vi "closeSine.vi"(8 "error in (no error)":errorcluster, 11 "VISA Refnum in":refnum<visa-resource-name>) -> (0 "error out":errorcluster)   [LabVIEW 2012]
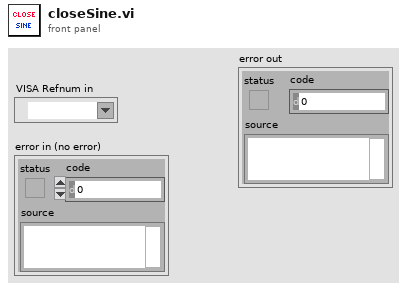
[diagram p1: front panel]
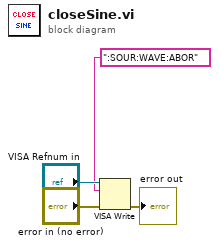
[diagram p0: block diagram]
diagram:
  n1 = VISA Write(VISA resource name="VISA Refnum in", write buffer=":SOUR:WAVE:ABOR", error in (no error)="error in (no error)") -> (error out=→"error out":errorcluster)  [unwired: 2 out]
